vi "Player Info.vi"(11 "Formics in":refnum<class "Formics.lvclass">) -> (1 "Victory Speech":string, 2 "Name":string, 3 "Formics out":refnum<class "Formics.lvclass">)   [LabVIEW 2015, in "Formics.lvclass"]
uses:
  Formics.lvclass
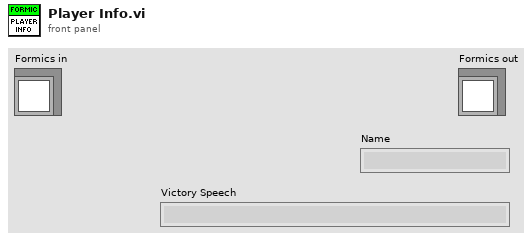
[diagram p1: front panel]
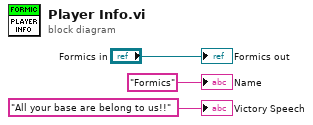
[diagram p0: block diagram]
diagram:
  "Formics out" <- "Formics in"
  "Name" <- "Formics" ("Name")
  "Victory Speech" <- "All your base are belong to us!!" ("Victory Speech")
